vi "Dateischreiben_Echtes_Signal_Simulation.vi"() -> ()   [LabVIEW 2016]
panel:
  out "PT":dbl
  out "Te":dbl
  in  "Messfrequenz":dbl=10.0
  in  "Spalten":string[](array[string])=["y-wert\n", "", "", ""]
  in  "Header":string[](array[string])=["Messlabor\n", "trajan_ursiwn", "21092023", "HTBLA Kaindorf"]
  out "Signalverlauf":dynamicdata(graph)
  in  "Eingangs-String":string="%f\\t%f\\t%f\\t%f\\t%f\\n"
  in  "Pfad":path=path "C:/Users/Messlabor_Kustos/Desktop/Schueler/4BHME/28.09.2023/DatenTabelleV2.xls"
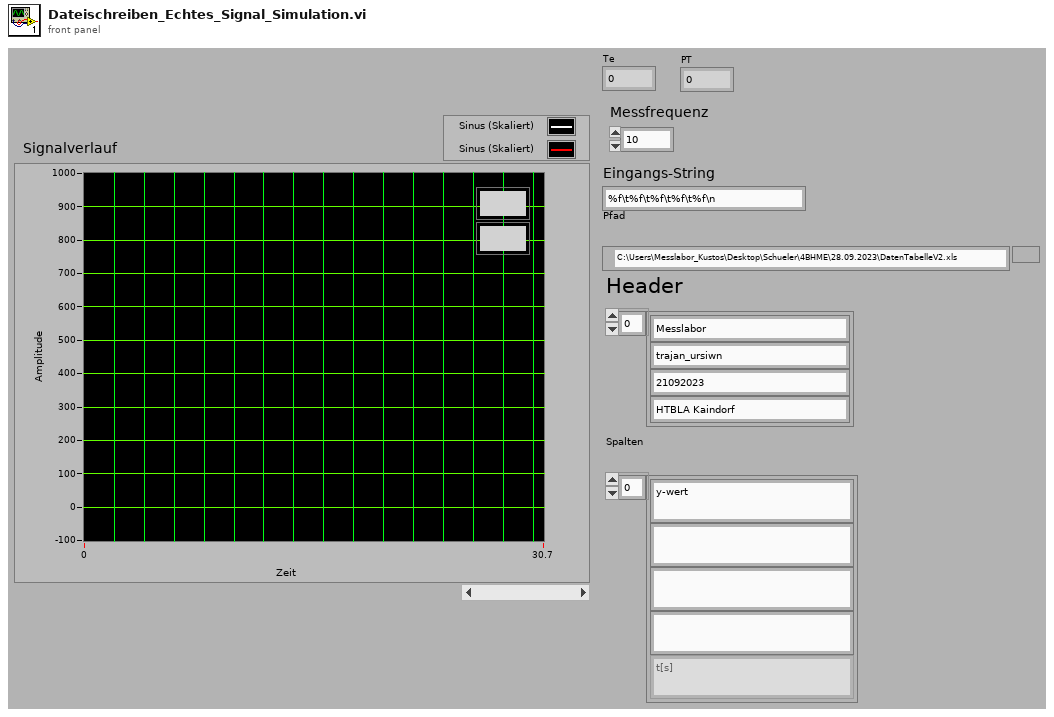
[diagram p1: front panel]
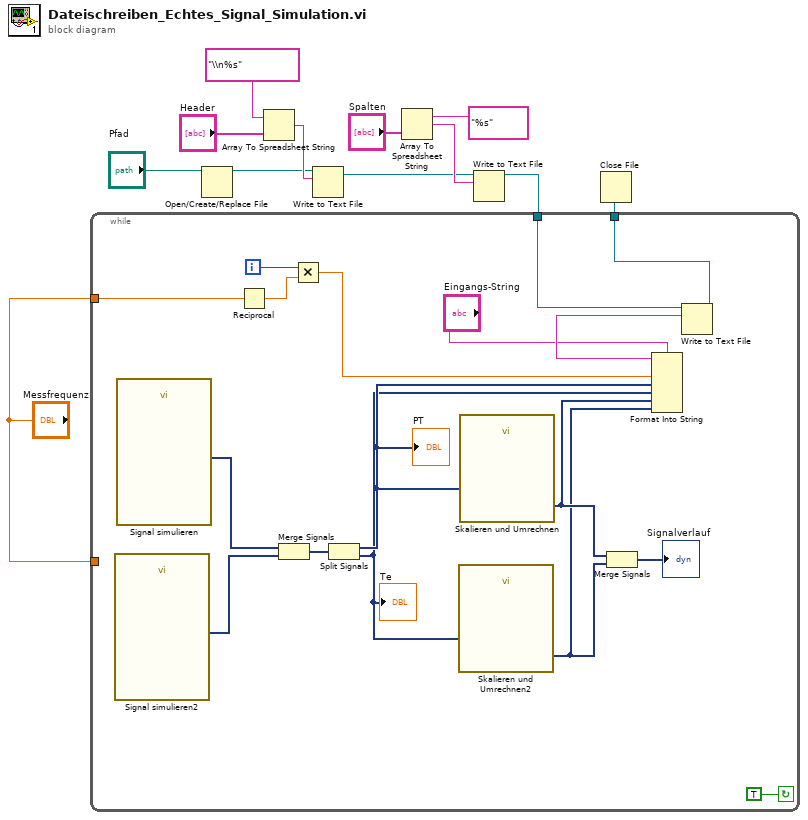
[diagram p0: block diagram]
diagram:
  n1 = Open/Create/Replace File(file path (use dialog)="Pfad") -> (refnum out=w4:refnum<file>)  [unwired: 5 in, 2 out]
  n2 = Array To Spreadsheet String(array="Header", 3:"\\n%s" ("Format-String")) -> (spreadsheet string=w6:string)  [unwired: 1 in]
  n3 = Write to Text File(file (use dialog)=w4, text=w6) -> (refnum out=w2:refnum<file>)  [unwired: 2 in, 2 out]
  n4 = Array To Spreadsheet String(array="Spalten", 3:"%s" ("Format-String")) -> (spreadsheet string=w5:string)  [unwired: 1 in]
  n5 = Write to Text File(file (use dialog)=w2, text=w5) -> (refnum out=w3:refnum<file>)  [unwired: 2 in, 2 out]
  n6 = while {
    tunnel: [w29] -> w12
    tunnel: w3 -> [w25]
    tunnel: "Messfrequenz" -> [w24]
    tunnel: "Messfrequenz" -> [_]
    i -> [w22]
    stop <- TRUE continue-if-true
    n7 = call "Signal simulieren2"() -> ("Sinus"=w19:dynamicdata)  [unwired: 14 in, 1 out]
    n8 = call "Signal simulieren"() -> ("Sinus"=w20:dynamicdata)  [unwired: 14 in, 1 out]
    n9 = Reciprocal(x=w24) -> (1/x=w23:dbl)
    n10 = Merge Signals(w20, w19) -> (w18:dynamicdata)
    n11 = Multiply(x=w22, y=w23) -> (x*y=w21:dbl)
    n12 = Split Signals(w18) -> (w16:dynamicdata, w15:dynamicdata)  [unwired: 2 in]
    "Te" <- w15
    "PT" <- w16
    n13 = call "Skalieren und Umrechnen2"("Signals"=w15) -> ("Scaled Signals"=w13:dynamicdata)  [unwired: 9 in, 1 out]
    n14 = call "Skalieren und Umrechnen"("Signals"=w16) -> ("Scaled Signals"=w14:dynamicdata)  [unwired: 9 in, 1 out]
    n15 = Merge Signals(w14, w13) -> (→"Signalverlauf":dynamicdata)
    n16 = Format Into String(format string="Eingangs-String", w21, w16, w15, w14, w13) -> (resulting string=w28:string)  [unwired: 2 in, 1 out]
    n17 = Write to Text File(file (use dialog)=w25, text=w28) -> (refnum out=w29:refnum<file>)  [unwired: 2 in, 2 out]
  }
  n18 = Close File(refnum=w12) -> ()  [unwired: 1 in, 2 out]
